vi "DS_NextStep.vi"(8 "error in (no error)":errorcluster, 10 "FromMyRiOtoUI":T1={"Accessibility"={"Command"=enum."End", "Error?"=FALSE, "Stop"=FALSE, "StopPomiar"=FALSE, "Name"="", "FilesPath"=path "", "ErrorHandler"={"Threads"=enum."Acquisistion", "ClearError"=FALSE, "Error Out "={"status"=FALSE, "code"=0, "source"=""}, "Error"=FALSE}, "Fs"=0.0}, "PropGraph"={"Raw Data"=[], "Poperties"={"RMS values"=[], "Max"=[], "Min"=[], "A(8)"=[], "t"=0.0, "A(8) Axis"=0.0, "Aw"=[], "Ak 30min"=0.0, "Ak_axis"=0, "Spec"=[]}, "Power Spectrum / PSD"=[]}, "No Data?"=FALSE, "WaveformData"=[]}, 11 "Previous step":T7) -> (0 "error out":errorcluster, 3 "Next Step":T7)   [LabVIEW 2019]
uses:
  TypeDef/#TypeDef_EnumOp_DataSaving.ctl
  Communication/TypeDef/#TypeDef_FromMRtoPC.ctl
  Communication/TypeDef/#TypeDef_FromPCtoMR.ctl
  Communication/TypeDef/#TypeDef_Command.ctl
  Communication/TypeDef/#TypeDef_ErrorHandler_prop.ctl
  Communication/TypeDef/#TypeDef_PropGraph.ctl
  Communication/TypeDef/#TypeDef_PropertiesToSave.ctl
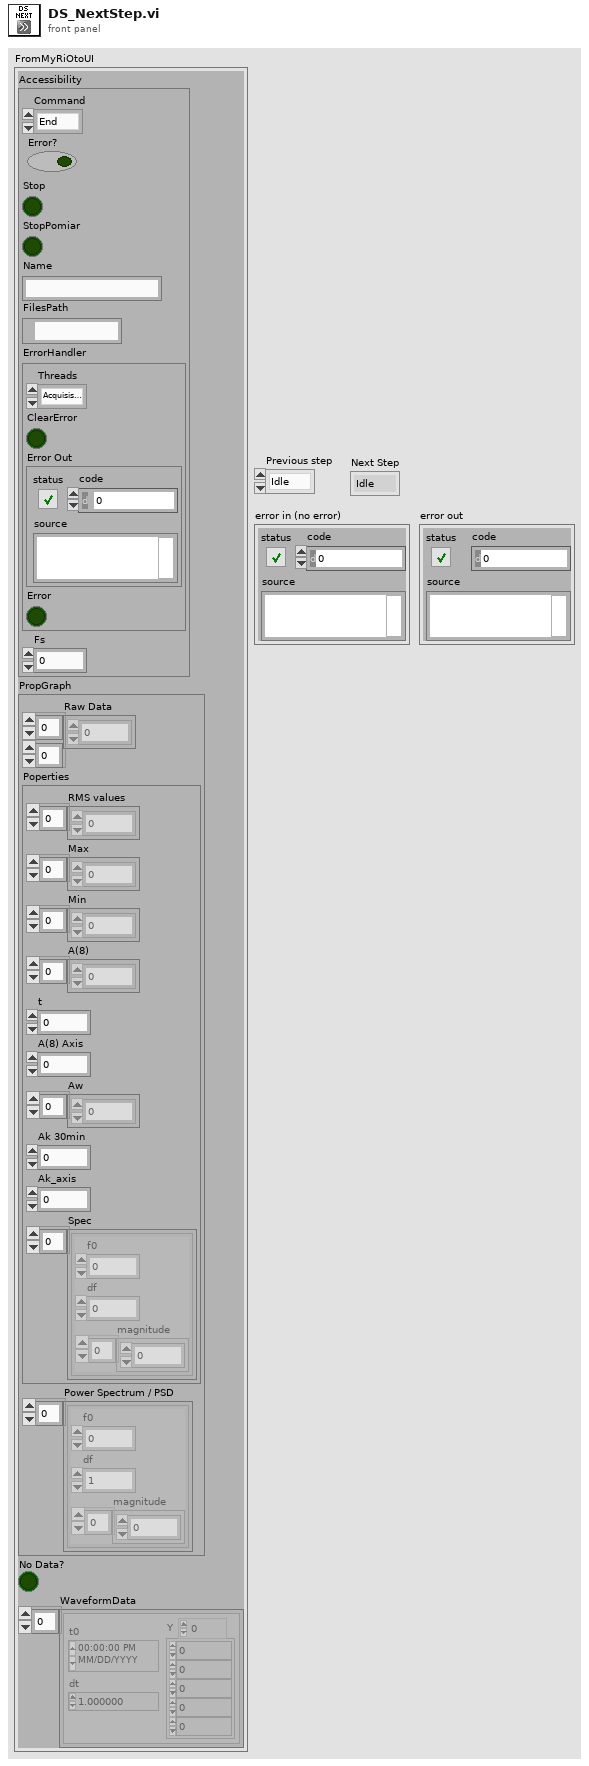
[diagram p1: front panel]
types:
  T1 = typedef "#TypeDef_FromMRtoPC.ctl" = cluster{"Accessibility":T2, "PropGraph":T5, "No Data?":bool, "WaveformData":waveform(dbl)[]}
  T2 = typedef "#TypeDef_FromPCtoMR.ctl" = cluster{"Command":T3, "Error?":bool, "Stop":bool, "StopPomiar":bool, "Name":string, "FilesPath":path, "ErrorHandler":T4, "Fs":dbl}
  T3 = typedef "#TypeDef_Command.ctl" = enum16{"Start", "End"}
  T4 = typedef "#TypeDef_ErrorHandler_prop.ctl" = cluster{"Threads":enum16{"Acquisistion", "Data Operation", "Save File"}, "ClearError":bool, "Error Out ":errorcluster, "Error":bool}
  T5 = typedef "#TypeDef_PropGraph.ctl" = cluster{"Raw Data":dbl[][], "Poperties":T6, "Power Spectrum / PSD":cluster{"f0":dbl, "df":dbl, "magnitude":dbl[]}[]}
  T6 = typedef "#TypeDef_PropertiesToSave.ctl" = cluster{"RMS values":dbl[], "Max":dbl[], "Min":dbl[], "A(8)":dbl[], "t":dbl, "A(8) Axis":dbl, "Aw":dbl[], "Ak 30min":dbl, "Ak_axis":i32, "Spec":cluster{"f0":dbl, "df":dbl, "magnitude":dbl[]}[]}
  T7 = typedef "#TypeDef_EnumOp_DataSaving.ctl" = enum16{"Idle", "Init", "Collecting", "Saving", "Deleting", "Error_Shutdown", "ClearError"}
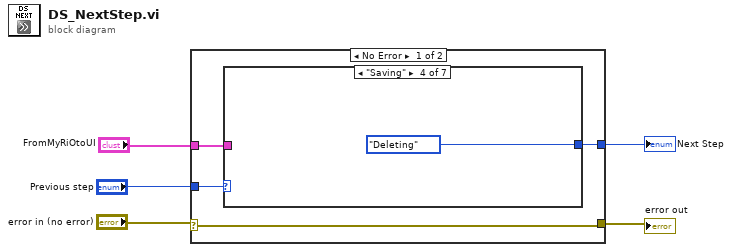
[diagram p0: block diagram]
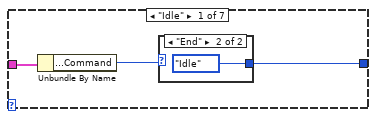
[diagram p2: hidden frame]
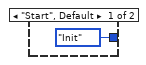
[diagram p3: hidden frame]
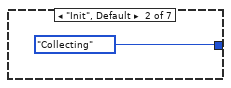
[diagram p4: hidden frame]
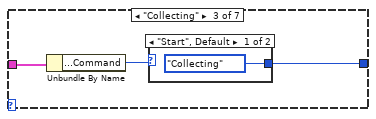
[diagram p5: hidden frame]
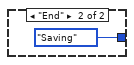
[diagram p6: hidden frame]
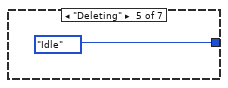
[diagram p7: hidden frame]
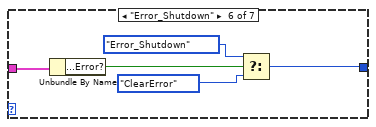
[diagram p8: hidden frame]
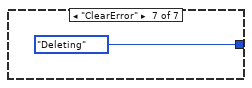
[diagram p9: hidden frame]
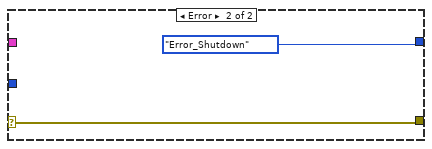
[diagram p10: hidden frame]
diagram:
  n1 = case shown="No Error" "error in (no error)" {
    selector: "error in (no error)" -> [w6 w30]
    tunnel: [w6 w30] -> w4
    tunnel: [w9 #TypeDef_EnumOp_DataSaving."Error_Shutdown" ("EnumOp_DataAcquisition")] -> w2
    tunnel: "FromMyRiOtoUI" -> [w8 _]
    tunnel: "Previous step" -> [w7 _]
    frame No Error {
      n2 = case shown="\"Saving\"" w7 {
        tunnel: w8 -> [w11 _ w17 _ _ w27 _]
        tunnel: [w10 #TypeDef_EnumOp_DataSaving."Collecting" ("EnumOp_DataAcquisition") w16 #TypeDef_EnumOp_DataSaving."Deleting" ("EnumOp_DataAcquisition") #TypeDef_EnumOp_DataSaving."Idle" ("EnumOp_DataAcquisition") w26 #TypeDef_EnumOp_DataSaving."Deleting" ("EnumOp_DataAcquisition")] -> w9
        frame "Idle" {
          n3 = Unbundle By Name(w11) -> ("Accessibility.Command"=w12:T3)
          n4 = case shown="\"End\"" w12 {
            tunnel: [#TypeDef_EnumOp_DataSaving."Init" ("EnumOp_DataAcquisition") #TypeDef_EnumOp_DataSaving."Idle" ("EnumOp_DataAcquisition")] -> w10
            frame "Start", Default {
            }
            frame "End" {
            }
          }
        }
        frame "Init", Default {
        }
        frame "Collecting" {
          n5 = Unbundle By Name(w17) -> ("Accessibility.Command"=w18:T3)
          n6 = case shown="\"Start\", Default" w18 {
            tunnel: [#TypeDef_EnumOp_DataSaving."Collecting" ("EnumOp_DataAcquisition") #TypeDef_EnumOp_DataSaving."Saving" ("EnumOp_DataAcquisition")] -> w16
            frame "Start", Default {
            }
            frame "End" {
            }
          }
        }
        frame "Saving" {
        }
        frame "Deleting" {
        }
        frame "Error_Shutdown" {
          n7 = Unbundle By Name(w27) -> ("Accessibility.Error?"=w25:bool)
          n8 = Select(t=#TypeDef_EnumOp_DataSaving."Error_Shutdown" ("EnumOp_DataAcquisition"), s=w25, f=#TypeDef_EnumOp_DataSaving."ClearError" ("EnumOp_DataAcquisition")) -> (s? t:f=w26:T7)
        }
        frame "ClearError" {
        }
      }
    }
    frame Error {
    }
  }
  "error out" <- w4
  "Next Step" <- w2
